vi "newlearn.vi"() -> ()   [LabVIEW 2013]
uses:
  <vilib>/LabVIEW Interface for Arduino/Type Defs/Pin Mode.ctl
  <vilib>/LabVIEW Interface for Arduino/Type Defs/Board Type.ctl
  <vilib>/LabVIEW Interface for Arduino/LabVIEW Interface for Arduino.lvlib
panel:
  in  "Value (0)":bool
  in  "Digital I/O Pin":u8
  in  "stop":bool
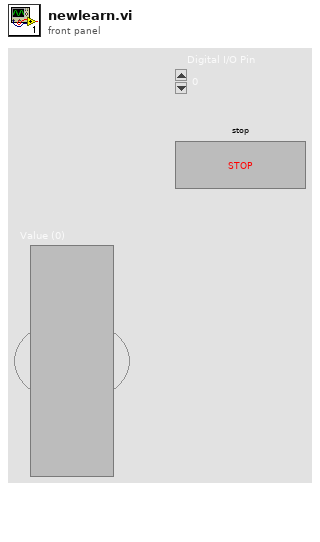
[diagram p1: front panel]
types:
  T1 = typedef "LabVIEW Interface for Arduino.lvlib/Board Type.ctl" = enum16{"Uno", "Dimuelanove w/Atmega 328", "Mega 2560"}
  T2 = typedef "LabVIEW Interface for Arduino.lvlib/Pin Mode.ctl" = enum8{"Input", "Output"}
  T3 = typedef "LabVIEW Interface for Arduino.lvlib/Arduino Resource.ctl" = cluster{"VISA resource":refnum<visa-resource-name>, "Board Type":T1, "Connection Type":enum8{"USB / Serial"}, "Bytes Per Packet (15)":u8}
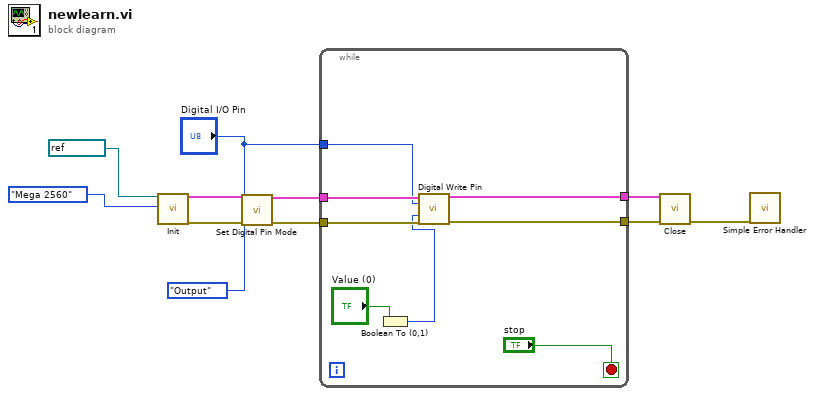
[diagram p0: block diagram]
diagram:
  n1 = call <vilib>:"Init.vi"("VISA resource"=refnum<visa-resource-name> "COM7", "Board Type (Uno)"=Board_Type."Mega 2560") -> ("Arduino Resource"=w9:T3, "error out"=w8:errorcluster)  [unwired: 16 in]
  n2 = call <vilib>:"Set Digital Pin Mode.vi"("Arduino Resource"=w9, "Digital I/O Pin"="Digital I/O Pin", "Pin Mode (Input)"=Pin_Mode."Output", "error in"=w8) -> ("Arduino Resource"=w11:T3, "error out"=w10:errorcluster)  [unwired: 10 in]
  n3 = while {
    tunnel: w11 -> [w18]
    tunnel: w10 -> [w17]
    tunnel: "Digital I/O Pin" -> [w16]
    tunnel: [w13] -> w5
    tunnel: [w12] -> w4
    stop <- "stop" stop-if-true
    n4 = Boolean To (0,1)(Boolean="Value (0)") -> (0, 1=w14:i16)
    n5 = call <vilib>:"Digital Write Pin.vi"("Arduino Resource"=w18, "Digital I/O Pin (0)"=w16, "Value (0)"=w14, "error in"=w17) -> ("Arduino Resource"=w13:T3, "error out"=w12:errorcluster)  [unwired: 10 in]
  }
  n6 = call <vilib>:"Close.vi"("Arduino Resource"=w5, "error in"=w4) -> ("error out"=w3:errorcluster)  [unwired: 13 in]
  n7 = call <vilib>:"Simple Error Handler.vi"("error in (no error)"=w3) -> ()  [unwired: 4 in, 5 out]
